vi "Aircraft 1.vi"(7 "Method":enum16{"Get", "Set"}(ring), 11 "Drone Information In":T1={"Aircraft ID"=0, "Tag ID"="", "System Status"="", "Base Mode"={"Custom Mode"=FALSE, "Test Enabled"=FALSE, "Autonomous Mode"=FALSE, "Guided Mode"=FALSE, "Stabilization Enabled"=FALSE, "HIL Enabled"=FALSE, "Manual Mode"=FALSE, "Arm"=FALSE}, "Armed/Disarmed"=FALSE, "Battery Voltage"=0.0, "Control Mode"=enum."Stabalise", "Initialisation"=0, "Coms with aircraft good"=FALSE, "Mode"="", "Mission Uploaded"=FALSE} {"Initialisation" scale=0.0..100.0}) -> (3 "Drone Information Out":T1={"Aircraft ID"=0, "Tag ID"="", "System Status"="", "Base Mode"={"Custom Mode"=FALSE, "Test Enabled"=FALSE, "Autonomous Mode"=FALSE, "Guided Mode"=FALSE, "Stabilization Enabled"=FALSE, "HIL Enabled"=FALSE, "Manual Mode"=FALSE, "Arm"=FALSE}, "Armed/Disarmed"=FALSE, "Battery Voltage"=0.0, "Control Mode"=enum."Stabalise", "Initialisation"=0, "Coms with aircraft good"=FALSE, "Mode"="", "Mission Uploaded"=FALSE} {"Initialisation" scale=0.0..100.0})   [LabVIEW 2014]
uses:
  Controls/Drone Information.ctl
  Controls/Base Mode.ctl
  Controls/Aircraft Mode.ctl
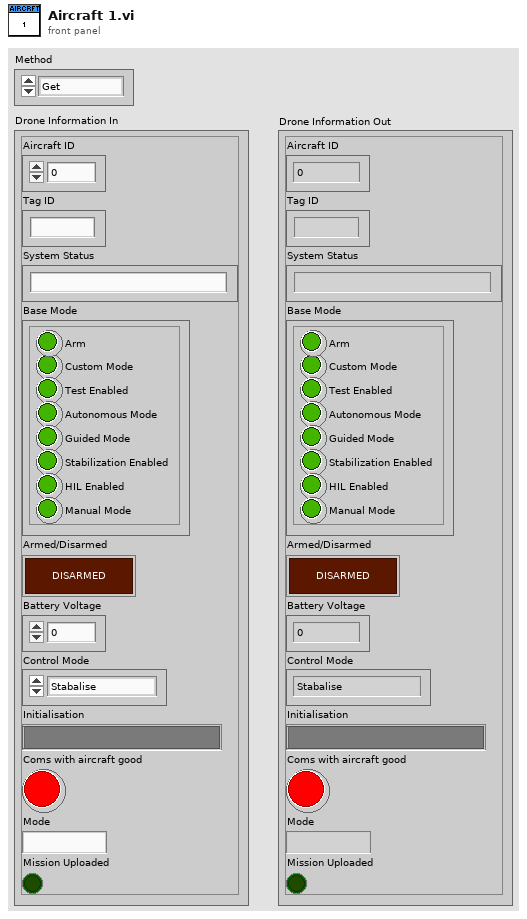
[diagram p1: front panel]
types:
  T1 = typedef "Drone Information.ctl" = cluster{"Aircraft ID":u8, "Tag ID":string, "System Status":string, "Base Mode":T2, "Armed/Disarmed":bool, "Battery Voltage":dbl, "Control Mode":T3, "Initialisation":u8, "Coms with aircraft good":bool, "Mode":string, "Mission Uploaded":bool}
  T2 = typedef "Base Mode.ctl" = cluster{"Custom Mode":bool, "Test Enabled":bool, "Autonomous Mode":bool, "Guided Mode":bool, "Stabilization Enabled":bool, "HIL Enabled":bool, "Manual Mode":bool, "Arm":bool}
  T3 = typedef "Aircraft Mode.ctl" = enum16{"Loiter", "Stabalise", "Failsafe", "Emergency Stop"}
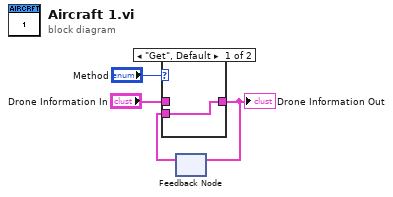
[diagram p0: block diagram]
diagram:
  n1 = feedback #1() -> (w1:T1)  [unwired: 1 in]
  n2 = case shown="\"Get\", Default" "Method" {
    tunnel: "Drone Information In" -> [_ w6]
    tunnel: [w5 w6] -> w2
    tunnel: w1 -> [w5 _]
    frame "Get", Default {
    }
    frame "Set" {
    }
  }
  "Drone Information Out" <- w2
  n3 = feedback-in #1(w2) -> ()
